vi "special spreadsheet.vi"(1 "input string":string) -> (0 "array":dbl[][](array[numeric]) format="%.2f")   [LabVIEW 2018]
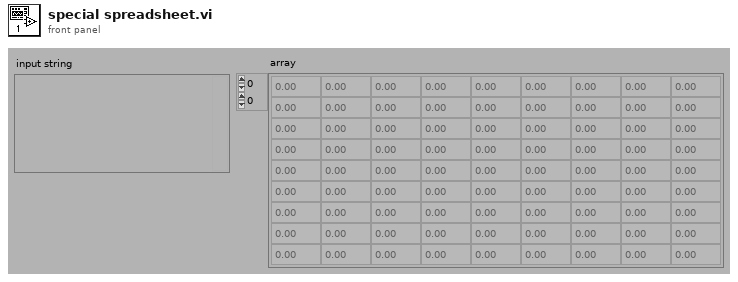
[diagram p1: front panel]
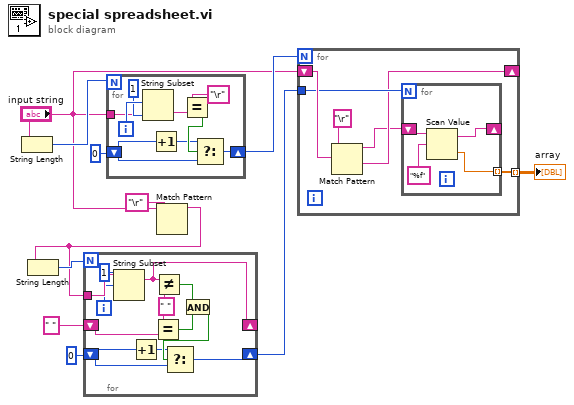
[diagram p0: block diagram]
diagram:
  n1 = String Length(string="input string") -> (length=w9:i32)
  n2 = for {
    N: w9 -> [_]
    tunnel: "input string" -> [w18]
    shift-right: [w12] -> w4
    shift-left: 0 -> [w14]
    i -> [w20]
    n3 = String Subset(string=w18, offset (0)=w20, length (rest)=1) -> (substring=w16:string)
    n4 = Increment(x=w14) -> (x+1=w13:i32)
    n5 = Equal?(x="\r", y=w16) -> (x = y?=w15:bool)
    n6 = Select(t=w13, s=w15, f=w14) -> (s? t:f=w12:i32)
  }
  n7 = Match Pattern(string="input string", regular expression="\r") -> (before substring=w7:string)  [unwired: 1 in, 3 out]
  n8 = String Length(string=w7) -> (length=w8:i32)
  n9 = for {
    N: w8 -> [_]
    tunnel: w7 -> [w23]
    shift-right: [w24] -> _
    shift-left: " " -> [w31]
    shift-right: [w25] -> w2
    shift-left: 0 -> [w26]
    i -> [w22]
    w32 = " "
    n10 = String Subset(string=w23, offset (0)=w22, length (rest)=1) -> (substring=w24:string)
    n11 = Increment(x=w26) -> (x+1=w27:i32)
    n12 = Equal?(x=w32, y=w31) -> (x = y?=w29:bool)
    n13 = Not Equal?(x=w24, y=w32) -> (x != y?=w30:bool)
    n14 = And(x=w30, y=w29) -> (x .and. y?=w28:bool)
    n15 = Select(t=w27, s=w28, f=w26) -> (s? t:f=w25:i32)
  }
  n16 = for {
    N: w4 -> [_]
    shift-right: [w34] -> _
    shift-left: "input string" -> [w37]
    tunnel: w2 -> [w36]
    tunnel: [w35] -> w1 mode=indexing
    n17 = Match Pattern(string=w37, regular expression="\r") -> (before substring=w33:string, after substring=w34:string)  [unwired: 1 in, 2 out]
    n18 = for {
      N: w36 -> [_]
      tunnel: [w40] -> w35 mode=indexing
      shift-right: [w41] -> _
      shift-left: w33 -> [w42]
      n19 = Scan Value(string=w42, format string="%f") -> (output string=w41:string, value=w40:dbl)  [unwired: 1 in]
    }
  }
  "array" <- w1
